vi "ryTimerEx.vi"() -> ()   [LabVIEW 2020]
uses:
  0042efe6-da2e-4d6a-bcc2-dcb81ee7ee9d.vi
  Lib/ryTimer.lvclass
panel:
  out "Last Ticks (ms)":u32
  out "Wait Time (ms)":u32
  out "Is Running?":bool
  out "Time Left (ms) [-1=Unknown]":i32
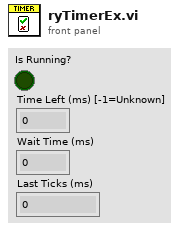
[diagram p1: front panel]
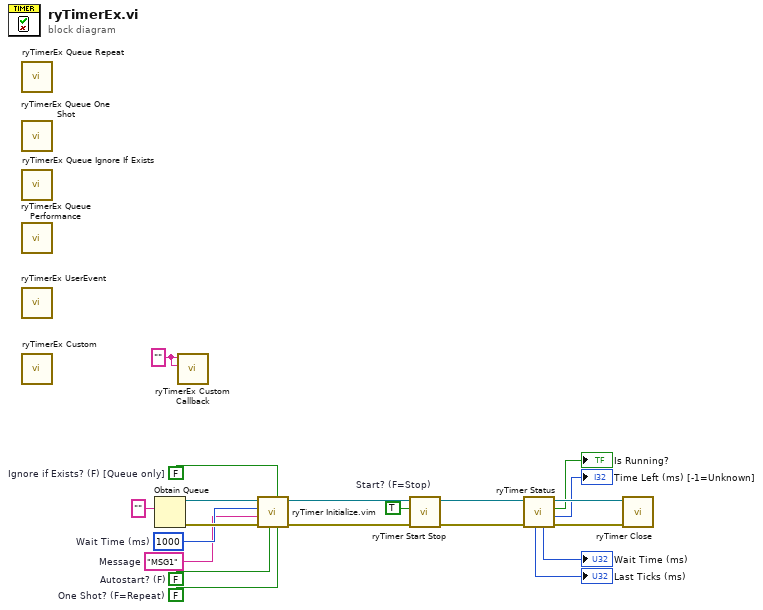
[diagram p0: block diagram]
diagram:
  w7 = FALSE  # Ignore if Exists? (F) [Queue only]
  w10 = TRUE  # Start? (F=Stop)
  w13 = FALSE  # One Shot? (F=Repeat)
  w15 = FALSE  # Autostart? (F)
  w16 = "MSG1"  # Message
  w17 = u32 1000  # Wait Time (ms)
  w20 = "" ("Destination Refnum")
  n1 = call "ryTimerEx Queue Repeat.vi"() -> ()  [unwired: 12 in]
  n2 = call "ryTimerEx Queue One Shot.vi"() -> ()  [unwired: 12 in]
  n3 = call "ryTimerEx Queue Ignore If Exists.vi"() -> ()  [unwired: 12 in]
  n4 = call "ryTimerEx Queue Performance.vi"() -> ()  [unwired: 12 in]
  n5 = call "ryTimerEx UserEvent.vi"() -> ()  [unwired: 12 in]
  n6 = call "ryTimerEx Custom.vi"() -> ()  [unwired: 12 in]
  n7 = Obtain Queue(element data type="") -> (queue out=w14:refnum<queue>, error out=w18:errorcluster)  [unwired: 4 in, 1 out]
  n8 = call "ryTimerEx Custom Callback.vi"("Message"=w20, "Destination Refnum"=w20) -> ()  [unwired: 10 in]
  n9 = call "ryTimer Initialize.vim"("One Shot? (F=Repeat)"=w13, "Ignore if Exists? (F) [Queue only]"=w7, "Autostart? (F)"=w15, "error in (no error)"=w18, "Message"=w16, "Wait Time (ms)"=w17, "Destination Refnum [Q,UE,Any]"=w14) -> ("error out"=w12:errorcluster, "Timer out"=w11:refnum<class "ryTimer.lvclass">)  [unwired: 3 in]
  n10 = call "ryTimer Start Stop.vi"("error in (no error)"=w12, "Start? (F=Stop)"=w10, "Timer in"=w11) -> ("error out"=w9:errorcluster, "Timer out"=w8:refnum<class "ryTimer.lvclass">)  [unwired: 7 in]
  n11 = call "ryTimer Status.vi"("error in (no error)"=w9, "Timer in"=w8) -> ("error out"=w6:errorcluster, "Time Left (ms) [-1=Unknown]"=→"Time Left (ms) [-1=Unknown]":i32, "Is Running?"=→"Is Running?":bool, "Timer out"=w5:refnum<class "ryTimer.lvclass">, "Wait Time (ms)"=→"Wait Time (ms)":u32, "Last Ticks (ms)"=→"Last Ticks (ms)":u32)  [unwired: 4 in]
  n12 = call "ryTimer Close.vi"("error in (no error)"=w6, "Timer in"=w5) -> ()  [unwired: 9 in, 1 out]
